vi "Create Puma560.vi"(8 "error in (no error)":errorcluster) -> (0 "error out":errorcluster, 3 "Puma560 Robot":refnum<class "NI_Robotics_Serial Robot Arm.lvclass">)   [LabVIEW 2017, in "NI_Kinematics.lvlib"]
uses:
  <vilib>/robotics/Kinematics/NI_Kinematics.lvlib
  <vilib>/robotics/Kinematics/Robot/NI_Robotics_Serial Robot Arm.lvclass
  <vilib>/robotics/Kinematics/Robot/Robot Pose.ctl
  <vilib>/robotics/Kinematics/Link/Joint Type.ctl
  <vilib>/robotics/Kinematics/Link/NI_Robotics_Link.lvclass
  <vilib>/Analysis/Matrix/Datatypes/RealMatrix.ctl
  <vilib>/Analysis/Matrix/NI_Matrix.lvlib
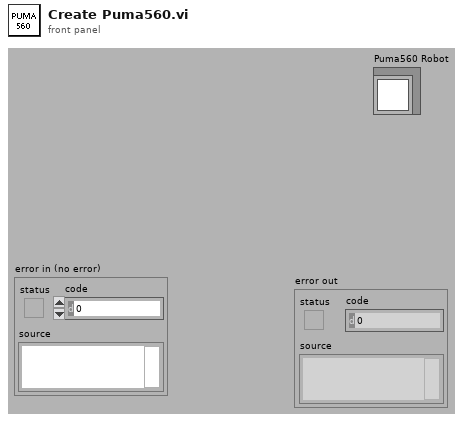
[diagram p1: front panel]
types:
  T1 = typedef "NI_Robotics_Link.lvclass/Joint Type.ctl" = enum16{"Revolute", "Prismatic"}
  T2 = cluster{"Twist Angle":dbl, "Length":dbl, "Rotation Angle":dbl, "Offset Distance":dbl, "Joint Type":T1, "Joint Coordinate Offset":dbl}
  T3 = cluster{"Twist Angle":dbl, "Length":dbl, "Rotation Angle":dbl, "Offset Distance":dbl, "Joint Type":T1, "Joint Coordinate Offset":dbl}[]
  T4 = typedef "NI_Robotics_Serial Robot Arm.lvclass/Robot Pose.ctl" = cluster{"name":string, "description":string, "joint positions":dbl[]}
  T5 = typedef "NI_Matrix.lvlib/RealMatrix.ctl" = dbl[][]
  T6 = cluster{"mass":dbl, "gear ratio":dbl, "motor inertia":dbl, "center of gravity":dbl[], "viscous friction":dbl, "positive coulomb friction":dbl, "negative coulomb friction":dbl, "inertia matrix":T5}
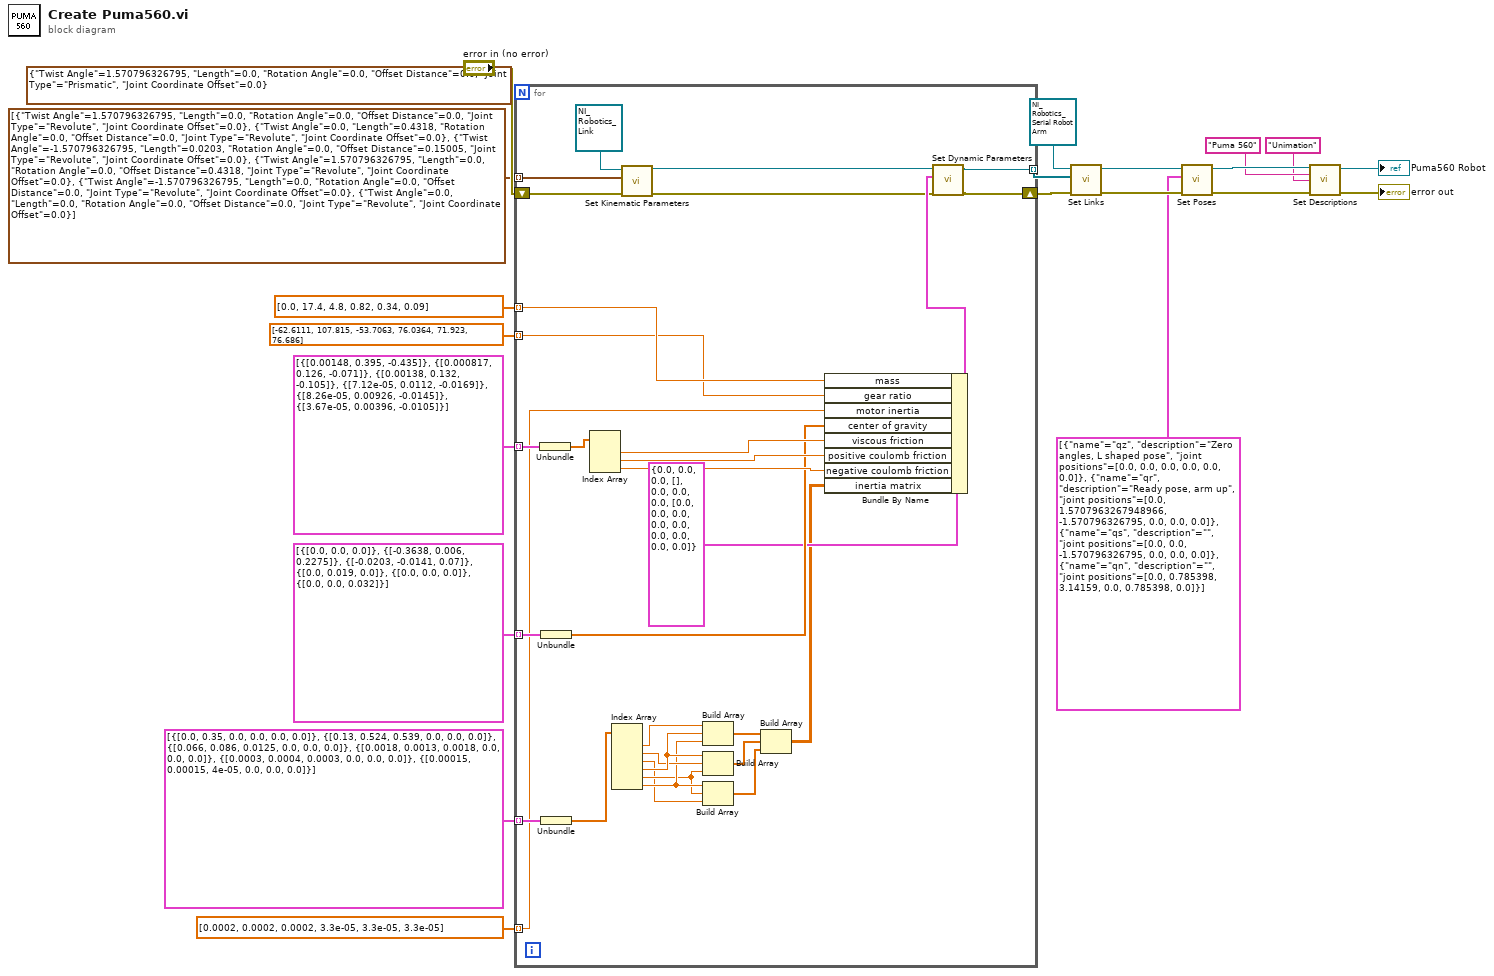
[diagram p0: block diagram]
diagram:
  (unwired) T2 {"Twist Angle"=1.570796326795, "Length"=0.0, "Rotation Angle"=0.0, "Offset Distance"=0.0, "Joint Type"=enum."Prismatic", "Joint Coordinate Offset"=0.0} ("Parameters")
  n1 = for {
    tunnel: T3 [{"Twist Angle"=1.570796326795, "Length"=0.0, "Rotation Angle"=0.0, "Offset Distance"=0.0, "Joint Type"=enum."Revolute", "Joint Coordinate Offset"=0.0}, {"Twist Angle"=0.0, "Length"=0.4318, "Rotation Angle"=0.0, "Offset Distance"=0.0, "Joint Type"=enum."Revolute", "Joint Coordinate Offset"=0.0}, {"Twist Angle"=-1.570796326795, "Length"=0.0203, "Rotation Angle"=0.0, "Offset Distance"=0.15005, "Joint Type"=enum."Revolute", "Joint Coordinate Offset"=0.0}, {"Twist Angle"=1.570796326795, "Length"=0.0, "Rotation Angle"=0.0, "Offset Distance"=0.4318, "Joint Type"=enum."Revolute", "Joint Coordinate Offset"=0.0}, {"Twist Angle"=-1.570796326795, "Length"=0.0, "Rotation Angle"=0.0, "Offset Distance"=0.0, "Joint Type"=enum."Revolute", "Joint Coordinate Offset"=0.0}, {"Twist Angle"=0.0, "Length"=0.0, "Rotation Angle"=0.0, "Offset Distance"=0.0, "Joint Type"=enum."Revolute", "Joint Coordinate Offset"=0.0}] -> [w46] mode=indexing
    tunnel: dbl[] [0.0, 17.4, 4.8, 0.82, 0.34, 0.09] -> [w44] mode=indexing
    tunnel: cluster{dbl[]}[] [{[0.0, 0.0, 0.0]}, {[-0.3638, 0.006, 0.2275]}, {[-0.0203, -0.0141, 0.07]}, {[0.0, 0.019, 0.0]}, {[0.0, 0.0, 0.0]}, {[0.0, 0.0, 0.032]}] -> [w51] mode=indexing
    tunnel: cluster{dbl[]}[] [{[0.0, 0.35, 0.0, 0.0, 0.0, 0.0]}, {[0.13, 0.524, 0.539, 0.0, 0.0, 0.0]}, {[0.066, 0.086, 0.0125, 0.0, 0.0, 0.0]}, {[0.0018, 0.0013, 0.0018, 0.0, 0.0, 0.0]}, {[0.0003, 0.0004, 0.0003, 0.0, 0.0, 0.0]}, {[0.00015, 0.00015, 4e-05, 0.0, 0.0, 0.0]}] -> [w50] mode=indexing
    tunnel: dbl[] [0.0002, 0.0002, 0.0002, 3.3e-05, 3.3e-05, 3.3e-05] -> [w38] mode=indexing
    tunnel: [w37] -> w13 mode=indexing
    shift-right: [w36] -> w14
    shift-left: "error in (no error)" -> [w47]
    tunnel: dbl[] [-62.6111, 107.815, -53.7063, 76.0364, 71.923, 76.686] -> [w43] mode=indexing
    tunnel: cluster{dbl[]}[] [{[0.00148, 0.395, -0.435]}, {[0.000817, 0.126, -0.071]}, {[0.00138, 0.132, -0.105]}, {[7.12e-05, 0.0112, -0.0169]}, {[8.26e-05, 0.00926, -0.0145]}, {[3.67e-05, 0.00396, -0.0105]}] -> [w49] mode=indexing
    n2 = Unbundle(w49) -> (w48:dbl[])
    n3 = Unbundle(w51) -> (w39:dbl[])
    n4 = Unbundle(w50) -> (w24:dbl[])
    n5 = Index Array(array=w48) -> (element #1=w42:dbl, element #2=w41:dbl, element #3=w40:dbl)  [unwired: 3 in]
    n6 = Index Array(array=w24) -> (element #1=w33:dbl, element #2=w31:dbl, element #3=w28:dbl, element #4=w32:dbl, element #5=w29:dbl, element #6=w30:dbl)  [unwired: 6 in]
    n7 = call <vilib>:"Set Kinematic Parameters.vi"("error in (no error)"=w47, "kinematic parameters"=w46, "link in"=refnum<class "NI_Robotics_Link.lvclass"> refnum ("Link")) -> ("error out"=w22:errorcluster, "link out"=w21:refnum<class "NI_Robotics_Link.lvclass">)  [unwired: 7 in]
    n8 = Build Array(w33, w32, w30) -> (w27:dbl[])
    n9 = Build Array(w32, w31, w29) -> (w26:dbl[])
    n10 = Build Array(w30, w29, w28) -> (w25:dbl[])
    n11 = Build Array(w27, w26, w25) -> (w23:dbl[][])
    n12 = Bundle By Name(cluster=T6 {"mass"=0.0, "gear ratio"=0.0, "motor inertia"=0.0, "center of gravity"=[], "viscous friction"=0.0, "positive coulomb friction"=0.0, "negative coulomb friction"=0.0, "inertia matrix"=[[0.0, 0.0, 0.0], [0.0, 0.0, 0.0], [0.0, 0.0, 0.0]]} ("dynamic parameters"), "mass"=w44, "gear ratio"=w43, "motor inertia"=w38, "center of gravity"=w39, "viscous friction"=w42, "positive coulomb friction"=w41, "negative coulomb friction"=w40, "inertia matrix"=w23) -> (w34:T6)
    n13 = call <vilib>:"Set Dynamic Parameters.vi"("error in (no error)"=w22, "dynamic parameters"=w34, "link in"=w21) -> ("error out"=w36:errorcluster, "link out"=w37:refnum<class "NI_Robotics_Link.lvclass">)  [unwired: 7 in]
  }
  n14 = call <vilib>:"Set Links.vi"("error in (no error)"=w14, "links"=w13, "serial arm in"=refnum<class "NI_Robotics_Serial Robot Arm.lvclass"> refnum ("Robot.lvclass")) -> ("error out"=w11:errorcluster, "serial arm out"=w12:refnum<class "NI_Robotics_Serial Robot Arm.lvclass">)  [unwired: 7 out]
  n15 = call <vilib>:"Set Poses.vi"("error in (no error)"=w11, "serial arm poses"=T4[] [{"name"="qz", "description"="Zero angles, L shaped pose", "joint positions"=[0.0, 0.0, 0.0, 0.0, 0.0, 0.0]}, {"name"="qr", "description"="Ready pose, arm up", "joint positions"=[0.0, 1.5707963267948966, -1.570796326795, 0.0, 0.0, 0.0]}, {"name"="qs", "description"="", "joint positions"=[0.0, 0.0, -1.570796326795, 0.0, 0.0, 0.0]}, {"name"="qn", "description"="", "joint positions"=[0.0, 0.785398, 3.14159, 0.0, 0.785398, 0.0]}] ("Poses"), "serial arm in"=w12) -> ("error out"=w8:errorcluster, "serial arm out"=w9:refnum<class "NI_Robotics_Serial Robot Arm.lvclass">)  [unwired: 7 out]
  n16 = call <vilib>:"Set Descriptions.vi"("Robot in"=w9, "Name"="Puma 560", "Manufacturer"="Unimation" ("Name"), "error in (no error)"=w8) -> ("Robot out"=→"Puma560 Robot":refnum<class "NI_Robotics_Serial Robot Arm.lvclass">, "error out"=→"error out":errorcluster)  [unwired: 10 in]
